vi "loadSettings.vi"(10 "This VI":refnum<vi>, 11 "Events and errors log":refnum<vi>) -> ()   [LabVIEW 2017]
panel:
  out "data":cluster{"Name":string, "Variant Data":variant}[](array[cluster])
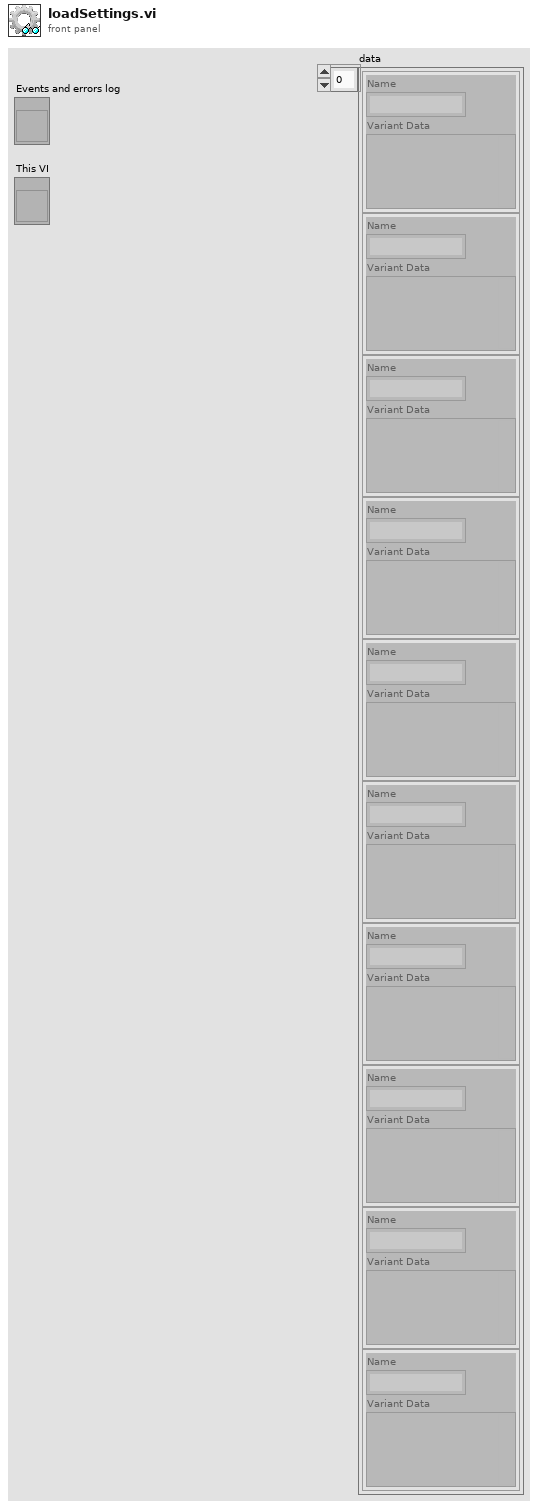
[diagram p1: front panel]
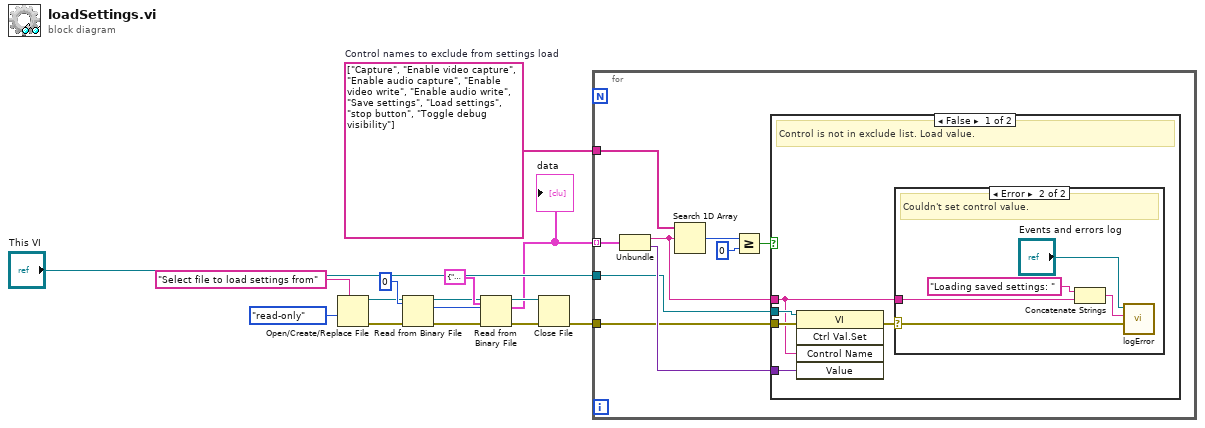
[diagram p0: block diagram]
diagram:
  w15 = string[] ["Capture", "Enable video capture", "Enable audio capture", "Enable video write", "Enable audio write", "Save settings", "Load settings", "stop button", "Toggle debug visibility"]  # Control names to exclude from settings load
  n1 = Open/Create/Replace File(prompt="Select file to load settings from", access (0:read/write)=enum16{"read/write", "read-only", "write-only"}."read-only") -> (refnum out=w2:refnum<file>, error out=w6:errorcluster)  [unwired: 4 in, 1 out]
  n2 = Read from Binary File(5:0 ("size(s)"), 8:w6, 11:w2) -> (0:w7:errorcluster, 2:w8:i32, 3:w3:refnum<file>)  [unwired: 3 in, 1 out]
  n3 = Read from Binary File(5:cluster{"Name":string, "Variant Data":variant} {"Name"="", "Variant Data"=variant}, 8:w7, 10:w8, 11:w3) -> (0:w13:errorcluster, 2:w10:cluster{"Name":string, "Variant Data":variant}[], 3:w12:refnum<file>)  [unwired: 2 in, 1 out]
  "data" <- w10
  n4 = Close File(refnum=w12, error in=w13) -> (error out=w14:errorcluster)  [unwired: 1 out]
  n5 = for {
    tunnel: w10 -> [w24] mode=indexing
    tunnel: "This VI" -> [w22]
    tunnel: w14 -> [w21]
    tunnel: w15 -> [w20]
    n6 = Unbundle(w24) -> ("Name"=w19:string, "Variant Data"=w23:variant)
    n7 = Search 1D Array(1D array=w20, element=w19) -> (index of element=w18:i32)  [unwired: 1 in]
    n8 = Greater Or Equal?(x=w18, y=0) -> (x >= y?=w16:bool)
    n9 = case shown="False" w16 {
      tunnel: w23 -> [w29 _]
      tunnel: w22 -> [w28 _]
      tunnel: w21 -> [w27 _]
      tunnel: w19 -> [w25 _]
      frame False {
        # "Control is not in exclude list. Load value."
        n10 = invoke class="VI" method="Ctrl Val.Set"(reference=w28, error in=w27, "Control Name"=w25, "Value"=w29) -> (error out=w26:errorcluster)  [unwired: 1 in, 4 out]
        n11 = case shown="Error" w26 {
          selector: w26 -> [_ w33]
          tunnel: w25 -> [_ w30]
          frame No Error {
          }
          frame Error {
            # "Couldn't set control value."
            n12 = Concatenate Strings("Loading saved settings: " ("Location"), w30) -> (w31:string)
            n13 = call "logError.vi"("Error to log"=w33, "Location"=w31, "Text reference"="Events and errors log") -> ()  [unwired: 8 in, 1 out]
          }
        }
      }
      frame True {
        # "Control is in exclude list. Do not retrieve saved value"
      }
    }
  }
